vi "Get Data from Icon Class.vi"(8 "error in (no error)":errorcluster, 11 "Icon in":refnum<class "Icon.lvclass">) -> (0 "error out":errorcluster, 1 "BW Image Data":T1, 2 "Color Image Data":T1, 3 "Icon data":T2={"Text Visible?"=FALSE, "Text Opacity"=0, "Templ Visible?"=FALSE, "Templ Opacity"=0, "Relative Path from 1 to 2"=path "", "Image"=bytes[0], "All User Layers"=[], "Body Text"={"Line 1 text"="", "Line 2 text"="", "Line 3 text"="", "Line 4 text"="", "Line 1 color"=0, "Line 2 color"=0, "Line 3 color"=0, "Line 4 color"=0, "Body Text Spec"={"Font"="", "Alignment"=0, "Size"=3}, "Center text vertically"=FALSE, "Capitalize Text"=FALSE}} {"Body Text"."Body Text Spec"."Alignment" items=["left", "center", "right"]})   [LabVIEW 2020, in "LabVIEW Icon API.lvlib"]
doc: "Extract data from the Icon class."
uses:
  <vilib>/LabVIEW Icon API/LabVIEW Icon API.lvlib
  <vilib>/LabVIEW Icon API/lv_icon/Controls/LabVIEW Icon Stored Information.ctl
  <vilib>/LabVIEW Icon API/lv_icon/Classes/Layer/Layer.lvclass
  <vilib>/LabVIEW Icon API/lv_icon/Controls/BodyText.ctl
  <vilib>/LabVIEW Icon API/lv_icon/Controls/Font.ctl
  <vilib>/LabVIEW Icon API/lv_icon/Controls/Alignment.ctl
  <vilib>/LabVIEW Icon API/lv_icon/Classes/Icon/Icon.lvclass
  <vilib>/picture/picture.llb/imagedata.ctl
  <vilib>/LabVIEW Icon API/lv_icon/Controls/Pathes.ctl
  <vilib>/LabVIEW Icon API/lv_icon/Classes/Icon Framework/Icon Framework.lvclass
  e:/builds/penguin/labview/branches/2020/dev/dist/vi.lib/LabVIEW Icon API/lv_icon/Classes/Layer/Layer.lvclass
  <vilib>/LabVIEW Icon API/lv_icon/lv_icon.lvlib
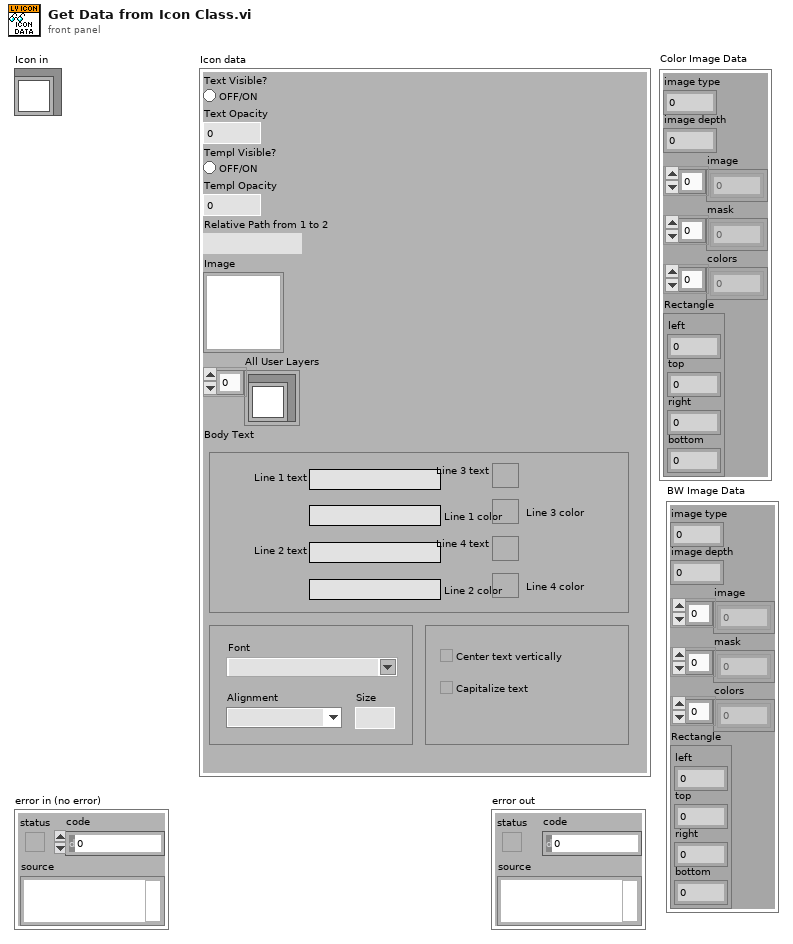
[diagram p1: front panel]
types:
  T1 = typedef "imagedata.ctl" = cluster{"image type":i32, "image depth":i32, "image":u8[], "mask":u8[], "colors":u32[], "Rectangle":cluster{"left":i16, "top":i16, "right":i16, "bottom":i16}}
  T2 = typedef "LabVIEW Icon Stored Information.ctl" = cluster{"Text Visible?":bool, "Text Opacity":u8, "Templ Visible?":bool, "Templ Opacity":u8, "Relative Path from 1 to 2":path, "Image":picture, "All User Layers":refnum<class "Layer.lvclass">[], "Body Text":T3}
  T3 = typedef "BodyText.ctl" = cluster{"Line 1 text":string, "Line 2 text":string, "Line 3 text":string, "Line 4 text":string, "Line 1 color":u32, "Line 2 color":u32, "Line 3 color":u32, "Line 4 color":u32, "Body Text Spec":cluster{"Font":T4, "Alignment":T5, "Size":u8}, "Center text vertically":bool, "Capitalize Text":bool}
  T4 = typedef "Font.ctl" = string
  T5 = typedef "Alignment.ctl" = u16
  T6 = typedef "Pathes.ctl" = enum16{"Root Path", "Icon Templates", "Icon Templates VI", "Icon Templates Lib", "Glyphs"}
  T7 = typedef "Layer.ctl" = cluster{"LayerIcon":picture, "LayerName":string, "Opacity":u8, "Visibility?":bool}
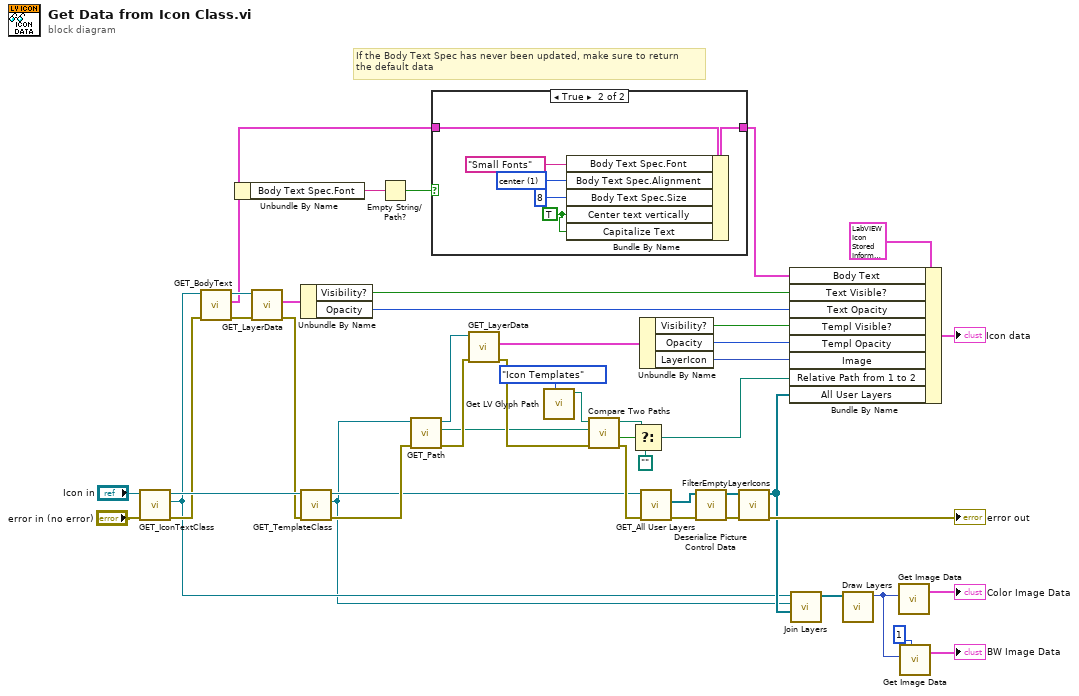
[diagram p0: block diagram]
diagram:
  # "If the Body Text Spec has never been updated, make sure to return\nthe default data"
  n1 = call-dynamic "GET_IconTextClass.vi"("error in (no error)"="error in (no error)", "Icon.lvclass in"="Icon in") -> ("error out"=w18:errorcluster, "Icon Framework.lvclass"=w9:refnum<class "Icon Framework.lvclass">, "Icon.lvclass out"=w27:refnum<class "Icon.lvclass">)  [unwired: 7 out]
  n2 = call-dynamic "GET_BodyText.vi"("error in (no error)"=w18, "Icon Framework.lvclass in"=w9) -> ("error out"=w22:errorcluster, "Body Text"=w4:T3, "Icon Framework.lvclass out"=w21:refnum<class "Icon Framework.lvclass">)  [unwired: 7 out]
  n3 = Unbundle By Name(w4) -> ("Body Text Spec.Font"=w2:T4)
  n4 = call-dynamic "GET_LayerData.vi"("error in (no error)"=w22, "Layer.lvclass in"=w21) -> ("error out"=w26:errorcluster, "Data"=w23:T7)  [unwired: 5 in, 3 out]
  n5 = Unbundle By Name(w23) -> ("Visibility?"=w24:bool, "Opacity"=w25:u8)
  n6 = call-dynamic "GET_TemplateClass.vi"("error in (no error)"=w26, "Icon.lvclass in"=w27) -> ("error out"=w38:errorcluster, "Icon Framework.lvclass"=w8:refnum<class "Icon Framework.lvclass">, "Icon.lvclass out"=w31:refnum<class "Icon.lvclass">)  [unwired: 7 in]
  n7 = Empty String/Path?(string/path=w2) -> (empty?=w1:bool)
  n8 = call <vilib>:"GET_Path.vi"("error in (no error)"=w38, "Icon Framework.lvclass in"=w8) -> ("error out"=w40:errorcluster, "Path"=w16:path, "Icon Framework.lvclass out"=w39:refnum<class "Icon Framework.lvclass">)  [unwired: 7 in]
  n9 = case shown="True" w1 {
    tunnel: w4 -> [w47 w53]
    tunnel: [w47 w51] -> w3
    frame False {
    }
    frame True {
      w48 = TRUE ("Center text vertically")
      w50 = T5 1 items=["left", "center", "right"] ("Body Text Spec.Alignment")
      n10 = Bundle By Name(cluster=w53, "Body Text Spec.Font"=T4 "Small Fonts", "Body Text Spec.Alignment"=w50, "Body Text Spec.Size"=u8 8, "Center text vertically"=w48, "Capitalize Text"=w48) -> (w51:T3)
    }
  }
  n11 = call-dynamic "GET_LayerData.vi"("error in (no error)"=w40, "Layer.lvclass in"=w39) -> ("error out"=w44:errorcluster, "Data"=w28:T7)  [unwired: 5 in, 3 out]
  n12 = call <vilib>:"Get LV Glyph Path.vi"("Path"=Pathes."Icon Templates") -> ("Requested Path"=w15:path)  [unwired: 2 in, 8 out]
  n13 = call <vilib>:"Compare Two Paths.vi"("error in (no error)"=w44, "Path 2"=w16, "Path 1"=w15) -> ("error out"=w42:errorcluster, "Path 2 Relative to Path 1?"=w36:bool, "Relative Path from 1 to 2"=w37:path)  [unwired: 6 out]
  n14 = Select(t=w37, s=w36, f=path "") -> (s? t:f=w41:path)
  n15 = Unbundle By Name(w28) -> ("Visibility?"=w29:bool, "Opacity"=w30:u8, "LayerIcon"=w5:picture)
  n16 = call-dynamic "GET_All User Layers.vi"("error in (no error)"=w42, "Icon.lvclass in"=w31) -> ("error out"=w32:errorcluster, "User Layer"=w33:refnum<class "Layer.lvclass">[])  [unwired: 7 in, 1 out]
  n17 = call <vilib>:"Deserialize Picture Control Data.vi"("error in (no error)"=w32, "Layers in"=w33) -> ("error out"=w35:errorcluster, "Layers out"=w34:refnum<class "Layer.lvclass">[])  [unwired: 8 out]
  n18 = call <vilib>:"FilterEmptyLayerIcons.vi"("error in (no error)"=w35, "Layers"=w34) -> ("error out"=→"error out":errorcluster, "Layers out"=w10:refnum<class "Layer.lvclass">[])  [unwired: 8 out]
  n19 = Bundle By Name(cluster=T2 {"Text Visible?"=FALSE, "Text Opacity"=0, "Templ Visible?"=FALSE, "Templ Opacity"=0, "Relative Path from 1 to 2"=path "", "Image"=bytes[0], "All User Layers"=[], "Body Text"={"Line 1 text"="", "Line 2 text"="", "Line 3 text"="", "Line 4 text"="", "Line 1 color"=0, "Line 2 color"=0, "Line 3 color"=0, "Line 4 color"=0, "Body Text Spec"={"Font"="", "Alignment"=0, "Size"=0}, "Center text vertically"=FALSE, "Capitalize Text"=FALSE}} ("Icon data"), "Body Text"=w3, "Text Visible?"=w24, "Text Opacity"=w25, "Templ Visible?"=w29, "Templ Opacity"=w30, "Image"=w5, "Relative Path from 1 to 2"=w41, "All User Layers"=w10) -> (→"Icon data":T2)
  n20 = call <vilib>:"Join Layers.vi"("User Layers"=w10, "Template"=w8, "Icon Text"=w9) -> ("Layer out"=w12:refnum<class "Layer.lvclass">[])  [unwired: 3 in, 5 out]
  n21 = call <vilib>:"Draw Layers.vi"("Layers"=w12) -> ("Picture"=w11:picture)  [unwired: 4 in, 6 out]
  n22 = call <vilib>:"Get Image Data.vi"("Pic In"=w11) -> ("image data out"=→"Color Image Data":T1)  [unwired: 2 in, 8 out]
  n23 = call <vilib>:"Get Image Data.vi"("depth (24)"=1 ("depth"), "Pic In"=w11) -> ("image data out"=→"BW Image Data":T1)  [unwired: 2 in, 7 out]
